vi "BSC203ConnectMoveTo.vi"() -> ()   [LabVIEW 2015]
uses:
  C:/Users/fmovagharnemati/OneDrive - THORLABS Inc/Desktop/Kinesis_with_LabVIEW_Examples_LV12 - v3/Thorlabs.MotionControl.Controls.dll
  Kinesis_with_LabVIEW_Examples_LV12 - v3/Thorlabs.MotionControl.Controls.dll
  C:/Users/fmovagharnemati/OneDrive - THORLABS Inc/Desktop/Kinesis_with_LabVIEW_Examples_LV12 - v3/Thorlabs.MotionControl.Benchtop.StepperMotorCLI.dll
  Kinesis_with_LabVIEW_Examples_LV12 - v3/Thorlabs.MotionControl.Benchtop.StepperMotorCLI.dll
panel:
  in  "?":bool
  in  "Set Abs Pos":bool
  in  "MoveAbsolute":bool
  in  "Home":bool
  in  "Abs Pos":dbl
  in  "Relative Move":bool
  in  "direction":i32(ring)=1 items=["Forward"=1, "Backward"=2]
  in  "Step Size":dbl
  in  "SerialNumber":string
  in  "ChannelNumber":i32
  in  "BenchtopStepperControl":refnum<k24>(container)
  # "Thorlabs Hardware: BSC20X -Benchtop Stepper Motor Controllers\nhttps://www.thorlabs.com/thorproduct.cfm?partnumber=BSC203\n\nDescription: This VI will enable you to communicate with BSC20X series to control stepper motors. \n\nInstructions: \n1) Connect your BSC20X  device to your PC & power the device, ensuring your stage/actutator is connected. For full device setup, the device product manual can be found on our website.\n2) Enter the device serial number as well as channel number below.\n4) Click 'Run' in the LabVIEW Toolbar which will attempt a connection, and enable the device.\n4) Ensure the device move path is clear for homing, and press Home.\n5) Await for device to be be available, and to have finished homing (Home indicator in control panel should be green).\n6) Input desired absolute position, and press 'Set Abs Pos' to set that for absolute moves.\n7) Similarly input desired direction and step size for relative moves.\n7) To end the Program click 'STOP'."
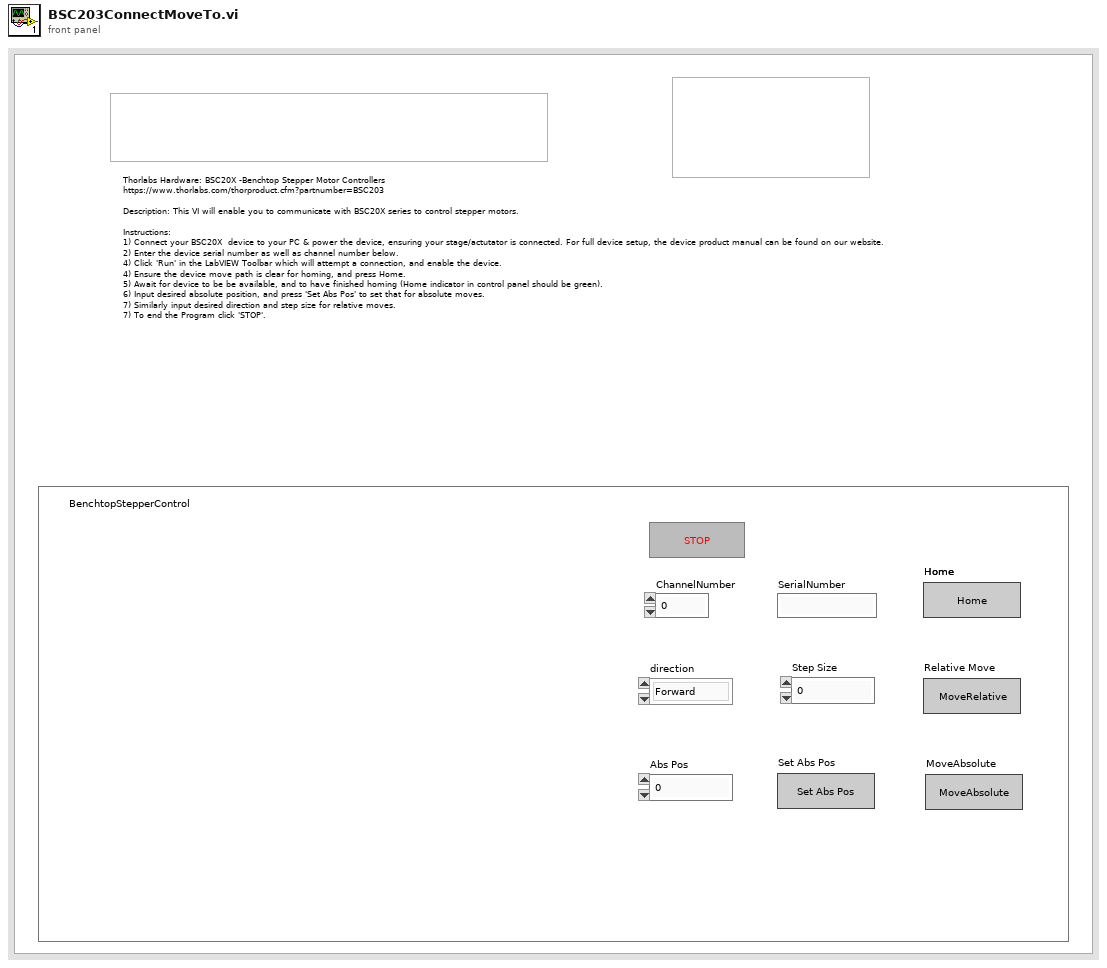
[diagram p1: front panel]
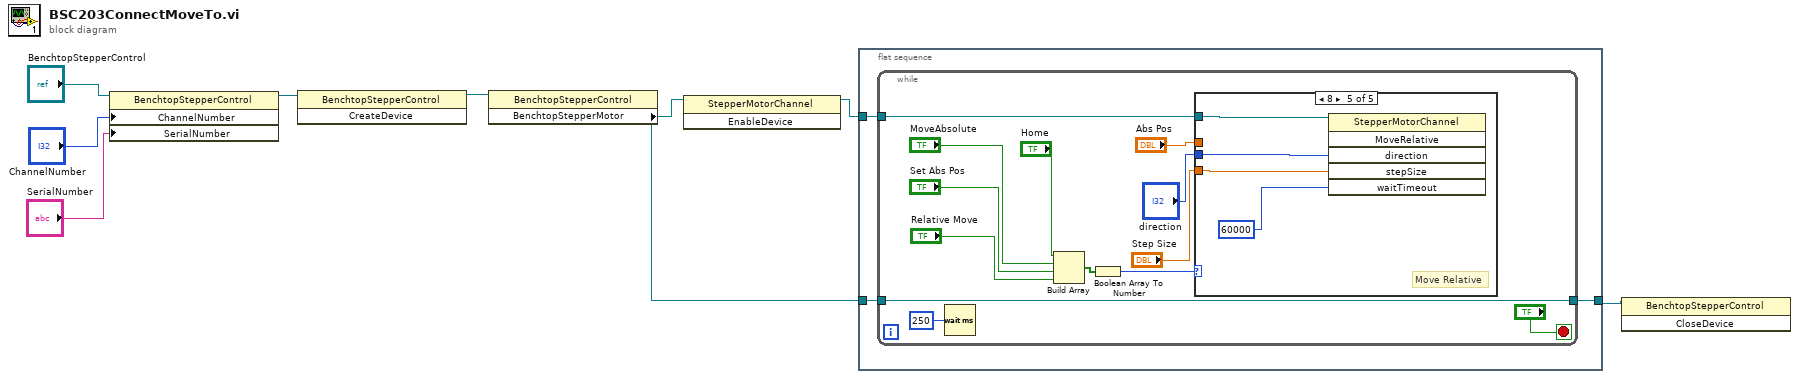
[diagram p0: block diagram]
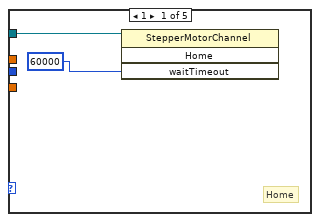
[diagram p2: hidden frame]
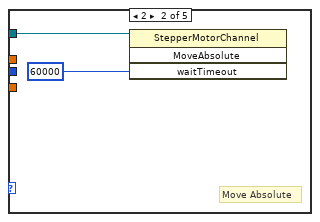
[diagram p3: hidden frame]
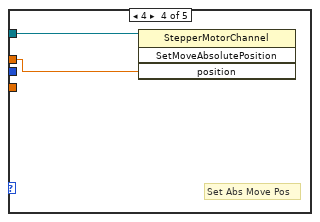
[diagram p5: hidden frame]
diagram:
  n1 = property class="BenchtopStepperControl"(reference="BenchtopStepperControl", "ChannelNumber"="ChannelNumber", "SerialNumber"="SerialNumber") -> (reference out=w6:refnum<k24>)  [unwired: 1 in, 1 out]
  n2 = invoke class="BenchtopStepperControl" method="CreateDevice"(reference=w6) -> (reference out=w5:refnum<k24>)  [unwired: 2 in, 2 out]
  n3 = property class="BenchtopStepperControl"(reference=w5) -> (reference out=w4:refnum<k24>, "BenchtopStepperMotor"=w2:refnum<k24>)  [unwired: 1 in, 1 out]
  n4 = invoke class="StepperMotorChannel" method="EnableDevice"(reference=w2) -> (reference out=w1:refnum<k24>)  [unwired: 2 in, 2 out]
  n5 = flat-sequence {
    tunnel: w4 -> [w12]
    tunnel: [w11] -> w3
    tunnel: w1 -> [w10]
    frame #0 {
      n6 = while {
        tunnel: [w17] -> w11
        tunnel: w10 -> [w21]
        tunnel: w12 -> [w17]
        stop <- "?" stop-if-true
        n7 = Wait (ms)(milliseconds to wait=u32 250) -> ()  [unwired: 1 out]
        n8 = Build Array("Home", "MoveAbsolute", "Set Abs Pos", "Relative Move") -> (w20:bool[])
        n9 = Boolean Array To Number(Boolean array=w20) -> (number=w19:u32)
        n10 = case shown="8" w19 {
          tunnel: w21 -> [w26 w28 _ w30 w33]
          tunnel: "Abs Pos" -> [_ _ _ w31 _]
          tunnel: "direction" -> [_ _ _ _ w34]
          tunnel: "Step Size" -> [_ _ _ _ w35]
          frame 1 {
            # "Home"
            n11 = invoke class="StepperMotorChannel" method="Home"(reference=w26, "waitTimeout"=60000) -> ()  [unwired: 2 in, 4 out]
          }
          frame 2 {
            # "Move Absolute"
            n12 = invoke class="StepperMotorChannel" method="MoveAbsolute"(reference=w28, "waitTimeout"=60000) -> ()  [unwired: 2 in, 4 out]
          }
          frame Default {
          }
          frame 4 {
            # "Set Abs Move Pos"
            n13 = invoke class="StepperMotorChannel" method="SetMoveAbsolutePosition"(reference=w30, "position"=w31) -> ()  [unwired: 2 in, 4 out]
          }
          frame 8 {
            # "Move Relative"
            n14 = invoke class="StepperMotorChannel" method="MoveRelative"(reference=w33, "direction"=w34, "stepSize"=w35, "waitTimeout"=60000) -> ()  [unwired: 2 in, 6 out]
          }
        }
      }
    }
  }
  n15 = invoke class="BenchtopStepperControl" method="CloseDevice"(reference=w3) -> ()  [unwired: 2 in, 3 out]
